vi "SendMotionPositions.vi"(8 "error in (no error)":errorcluster, 9 "Axis Position, eng.":dbl, 10 "mmWave Axis Name":string, 11 "SendMessage in":refnum<class "SendMessage.lvclass">) -> (0 "error out":errorcluster, 3 "SendMessage out":refnum<class "SendMessage.lvclass">)   [LabVIEW 2018, in "SendMessage.lvclass"]
uses:
  SendMessage.lvclass
  Support/MessageAPI/UIMessage.ctl
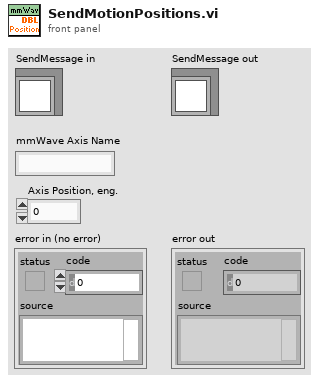
[diagram p1: front panel]
types:
  T1 = typedef "UIMessage.ctl" = cluster{"EventCode":i32, "Numeric":dbl, "String":string, "Variant":variant}
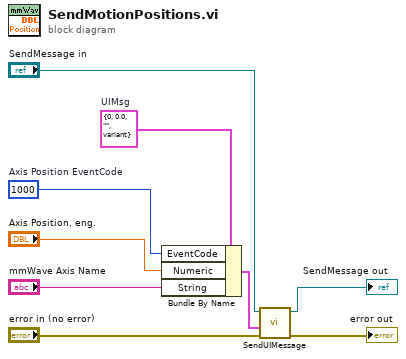
[diagram p0: block diagram]
diagram:
  w3 = T1 {"EventCode"=0, "Numeric"=0.0, "String"="", "Variant"=variant}  # UIMsg
  w1 = 1000  # Axis Position EventCode
  n1 = Bundle By Name(cluster=w3, "EventCode"=w1, "Numeric"="Axis Position, eng.", "String"="mmWave Axis Name") -> (w2:T1)
  n2 = call-dynamic "SendUIMessage.vi"("error in (no error)"="error in (no error)", "UIMsg"=w2, "SendMessage in"="SendMessage in") -> ("error out"=→"error out":errorcluster, "SendMessage out"=→"SendMessage out":refnum<class "SendMessage.lvclass">)  [unwired: 7 in]
